vi "VLF_draw.vi"(8 "Trial_Number":i32=1, 11 "HRV(VLF, LF, HF, PPI)":path) -> (3 "Icon1":dbl[][](graph))   [LabVIEW 2014]
uses:
  <vilib>/Utility/file.llb/Read From Spreadsheet File (DBL).vi
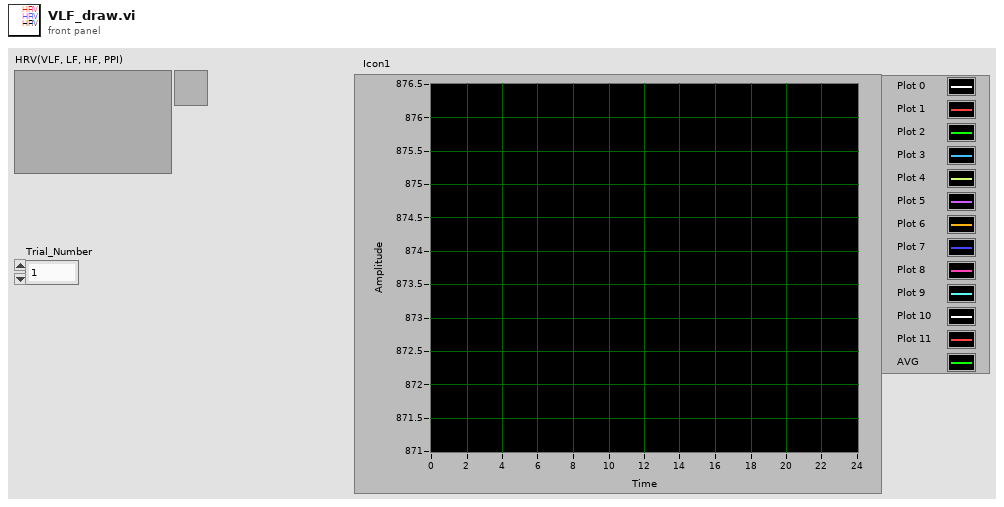
[diagram p1: front panel]
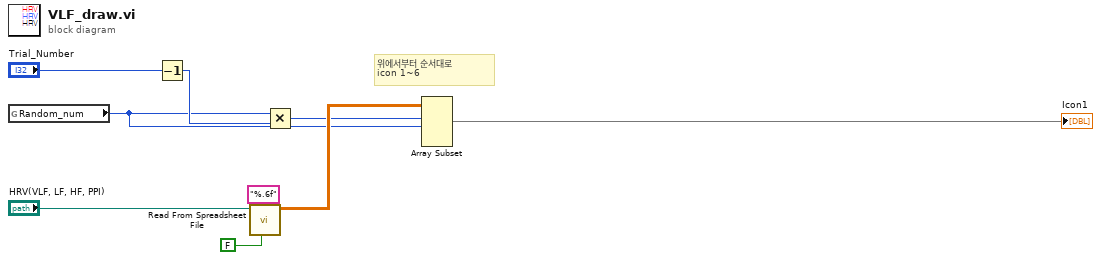
[diagram p0: block diagram]
diagram:
  # "위에서부터 순서대로 \nicon 1~6"
  n1 = global read "Control_Panel.vi" "Random_num"() -> (w2:i32)
  n2 = Decrement(x="Trial_Number") -> (x-1=w4:i32)
  n3 = call-poly <vilib>:"Read From Spreadsheet File.vi"("transpose (no:F)"=FALSE, "format (%.3f)"="%.6f", "file path (dialog if empty)"="HRV(VLF, LF, HF, PPI)") -> ("all rows"=w5:dbl[][])  [unwired: 4 in, 4 out]
  n4 = Multiply(x=w2, y=w4) -> (x*y=w3:i32)
  n5 = Array Subset(array=w5, index (row)=w3, length (row)=w2) -> (→"Icon1":dbl[][])  [unwired: 2 in]
